vi "TIC_main.vi"() -> ()   [LabVIEW 2011]
panel:
  out "dT/dt (K / min)":dbl
  in  "setPID":bool
  in  "D":dbl
  in  "I":dbl
  in  "P":dbl
  out "Ramp in K/s":dbl
  out "Waveform Chart":dbl(graph)
  out "Ramp T (K)":dbl
  out "OldVal":dbl
  in  "Ramp (K/min)":dbl
  in  "Setpoint (K)":dbl
  in  "TIC 500":refnum<visa-resource-name>="COM6"
  out "stateMachine0":string
  in  "EXIT":bool
  in  "Valve open(V)":dbl min=0.0 max=10.0 step=0.05
  out "Valve (V)":dbl format="%.1g"
  out "Heater OUT (W)":dbl
  out "Temperature (K)":dbl
  # "T > N2: P I D\n2.064  0.016   40.516"
  # "HELIUM: P I D\n0.753  0.024   4.154"
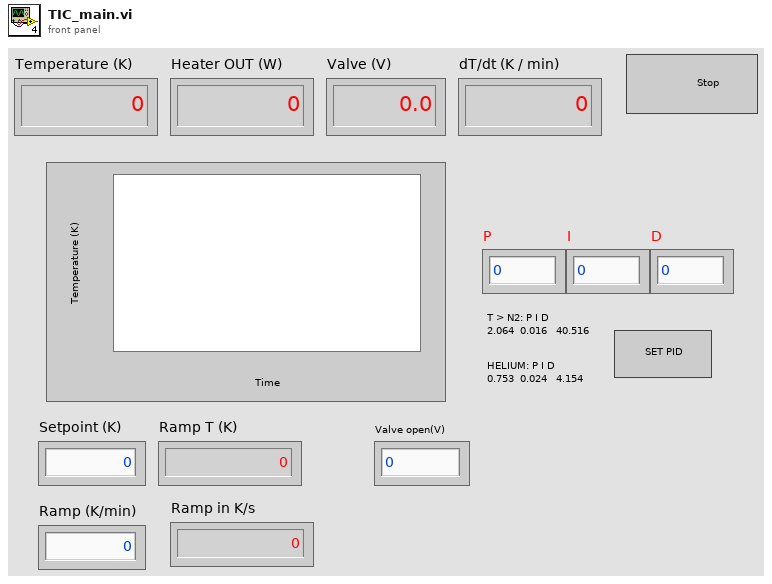
[diagram p1: front panel]
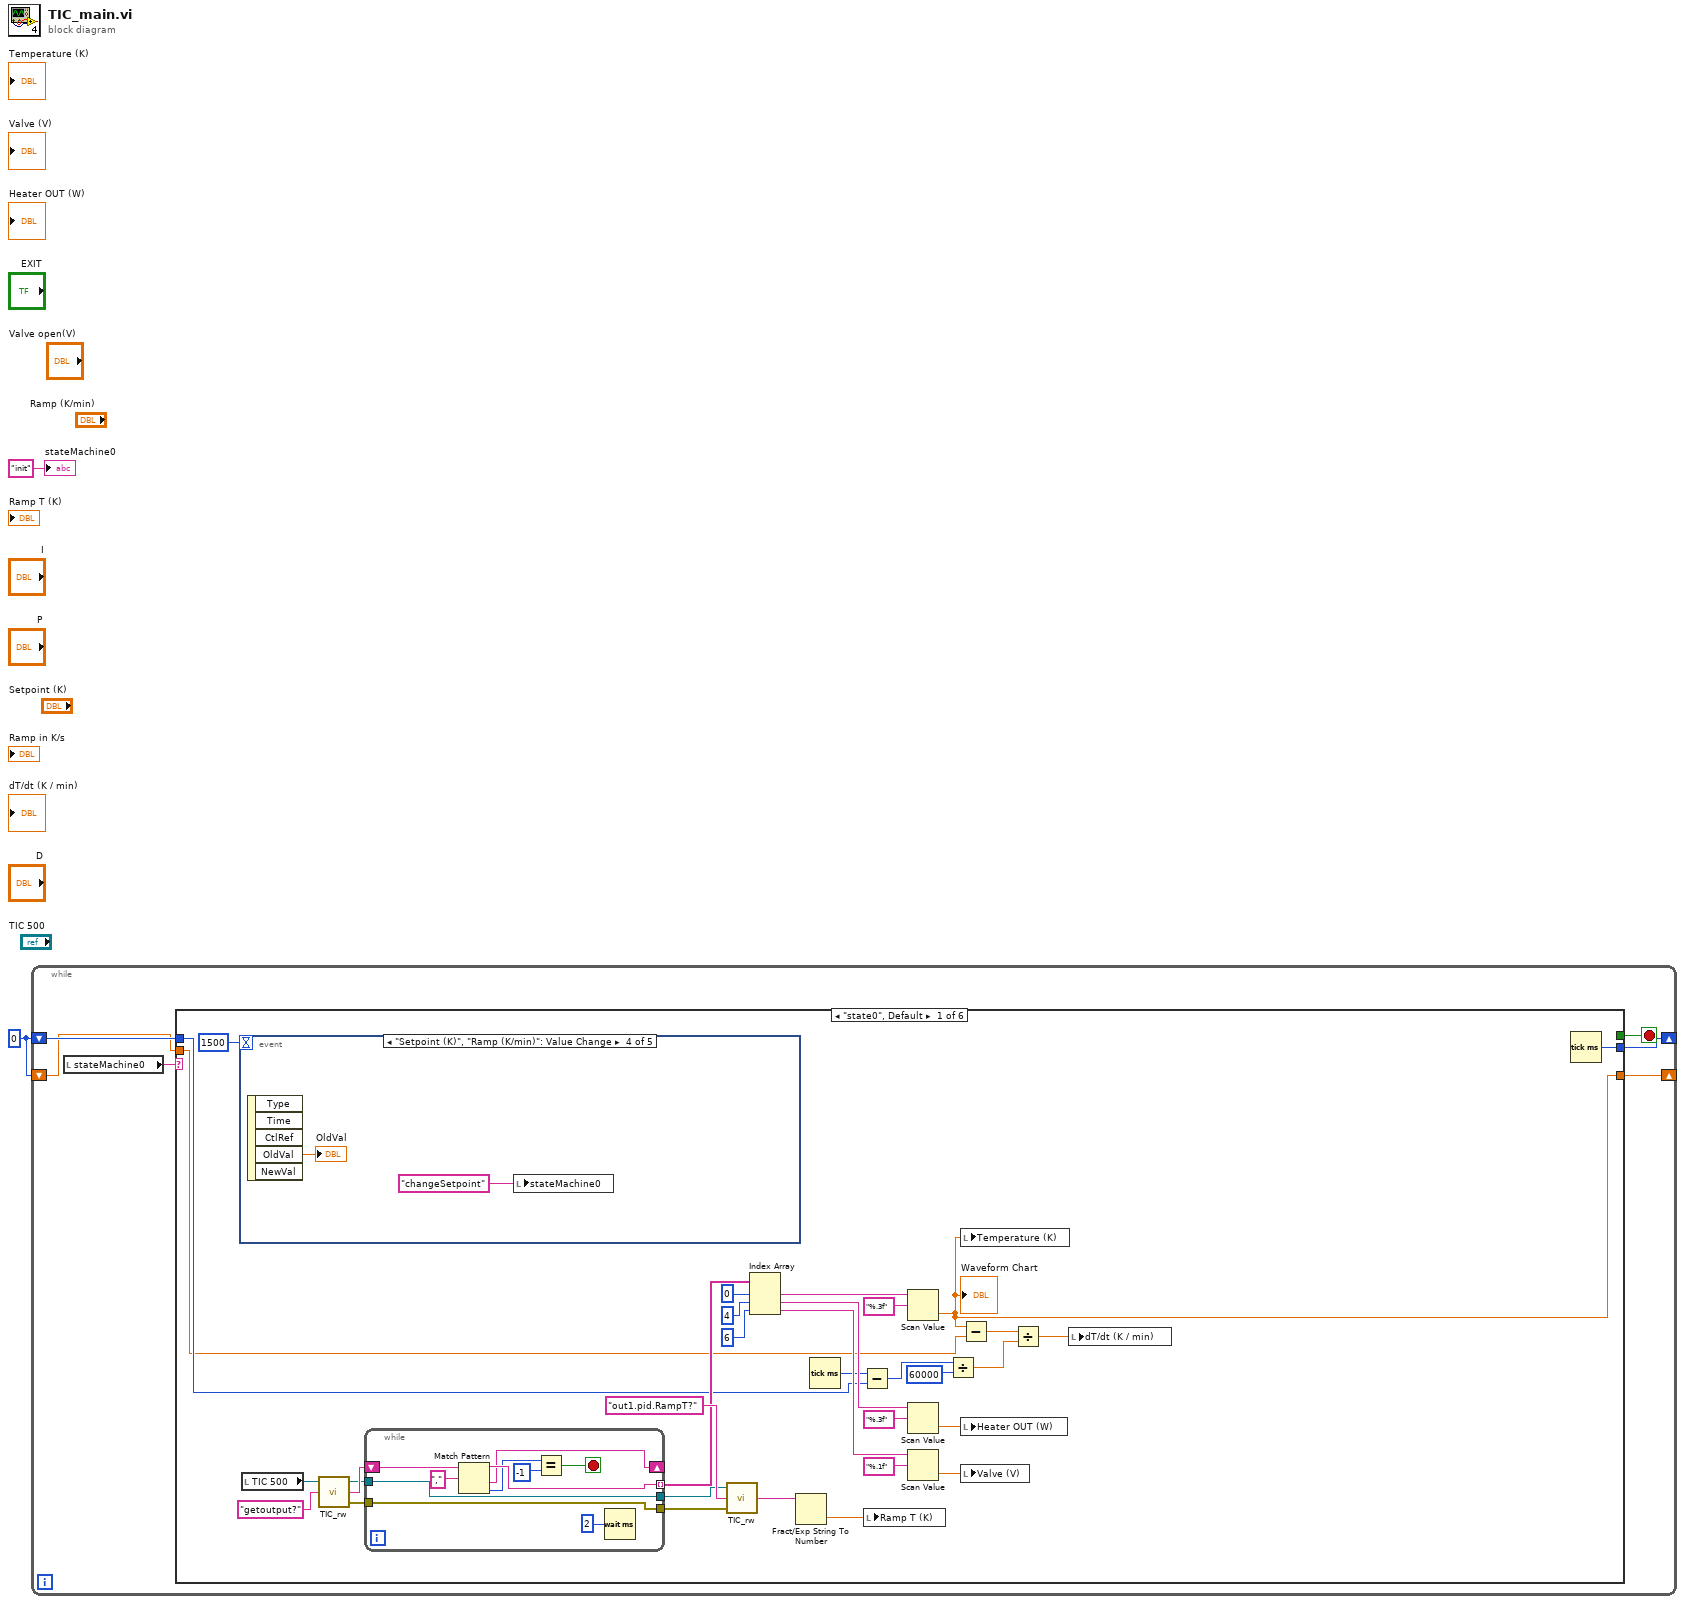
[diagram p0: block diagram]
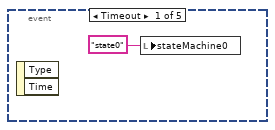
[diagram p2: hidden frame]
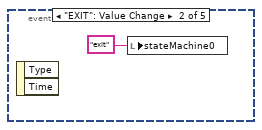
[diagram p3: hidden frame]
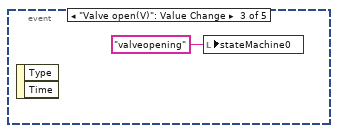
[diagram p4: hidden frame]
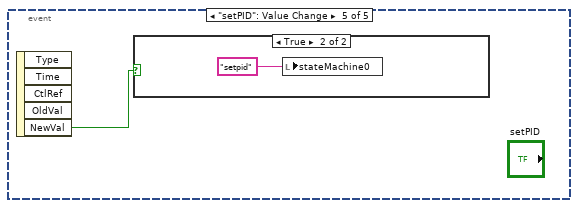
[diagram p5: hidden frame]
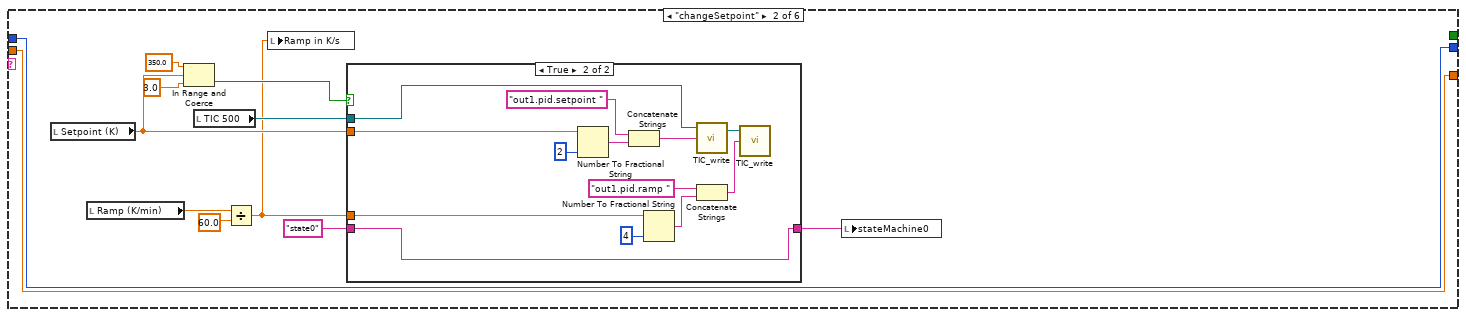
[diagram p7: hidden frame]
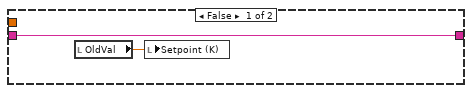
[diagram p8: hidden frame]
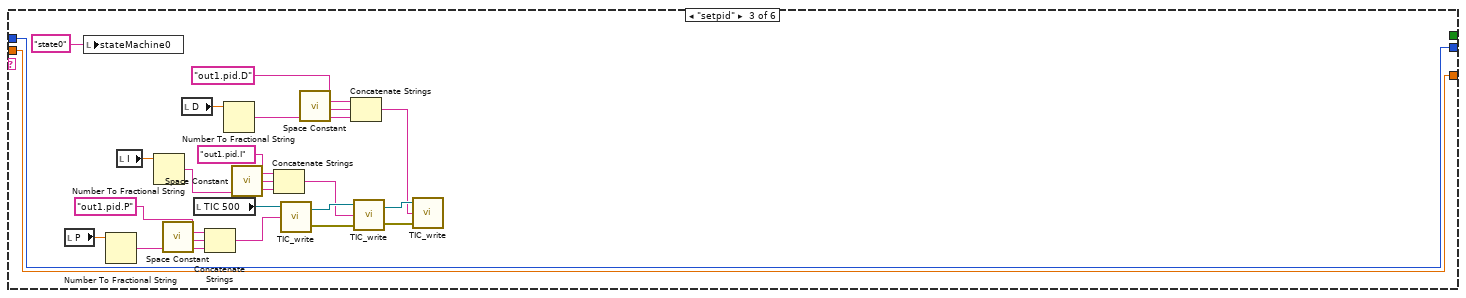
[diagram p9: hidden frame]
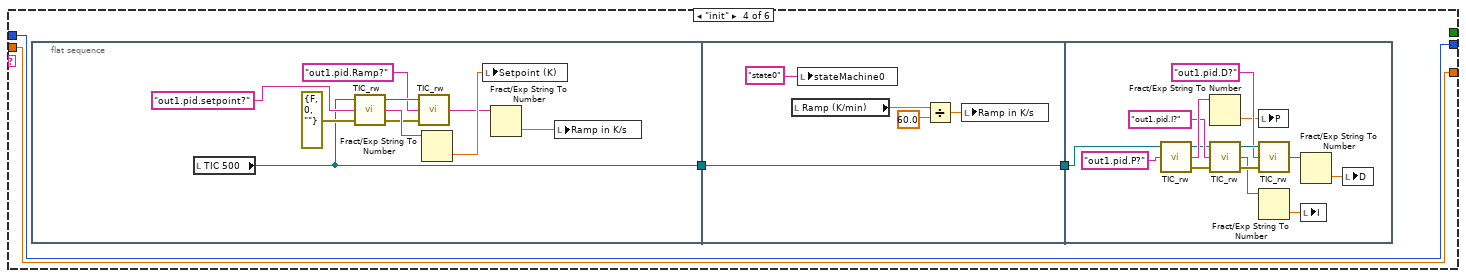
[diagram p10: hidden frame]
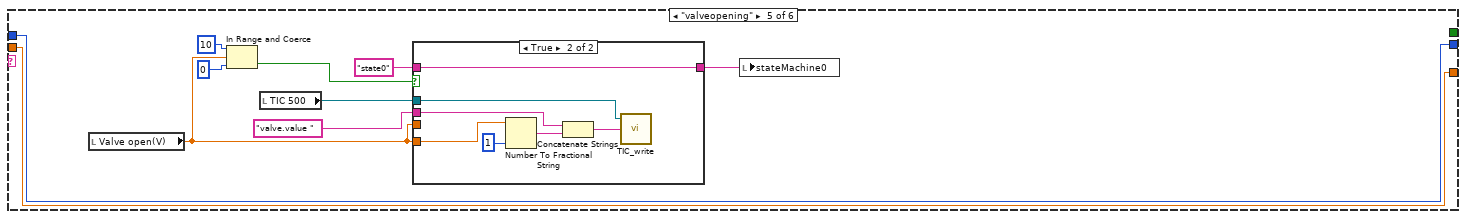
[diagram p11: hidden frame]
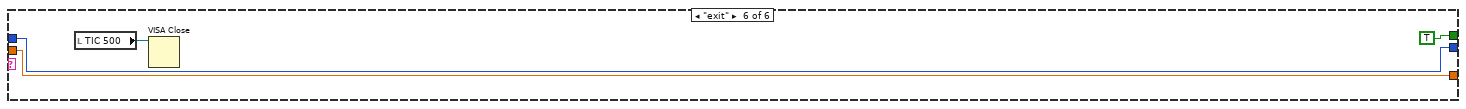
[diagram p13: hidden frame]
diagram:
  w1 = u32 0 ("millisecond timer value")
  n1 = while {
    shift-right: [w6] -> _
    shift-left: w1 -> [w5]
    shift-right: [w4] -> _
    shift-left: w1 -> [w3]
    stop <- w7 stop-if-true
    n2 = local read "stateMachine0"() -> (w8:string)
    n3 = case shown="\"state0\", Default" w8 {
      tunnel: [_ _ _ _ _ TRUE] -> w7
      tunnel: [w18 w60 w87 w109 w143 w161] -> w6
      tunnel: w5 -> [w16 w60 w87 w109 w143 w161]
      tunnel: [w10 w59 w86 w110 w142 w160] -> w4
      tunnel: w3 -> [w9 w59 w86 w110 w142 w160]
      frame "state0", Default {
        n4 = event shown="[3] \"Setpoint (K)\", \"Ramp (K/min)\": Value Change" {
          selector: _ -> [_ _ _ _ _]
          dyn-events: _ -> [_ _ _ _ _]
          timeout: 1500 -> [_ _ _ _ _]
          event Timeout {
            n5 = event-data() -> ()  [unwired: 1 in, 2 out]
            n6 = local write "stateMachine0"("state0") -> ()
          }
          event "EXIT": Value Change {
            n7 = event-data() -> ()  [unwired: 1 in, 2 out]
            n8 = local write "stateMachine0"("exit") -> ()
          }
          event "Valve open(V)": Value Change {
            n9 = event-data() -> ()  [unwired: 1 in, 2 out]
            n10 = local write "stateMachine0"("valveopening") -> ()
          }
          event "Setpoint (K)", "Ramp (K/min)": Value Change {
            n11 = event-data() -> ("OldVal"=→"OldVal":dbl)  [unwired: 1 in, 4 out]
            n12 = local write "stateMachine0"("changeSetpoint") -> ()
          }
          event "setPID": Value Change {
            n13 = event-data() -> ("NewVal"=w57:bool)  [unwired: 1 in, 4 out]
            n14 = case shown="True" w57 {
              frame False {
              }
              frame True {
                n15 = local write "stateMachine0"("setpid") -> ()
              }
            }
          }
        }
        n16 = local read "TIC 500"() -> (w40:refnum<visa-resource-name>)
        n17 = call "TIC_rw.vi"("write buffer"="getoutput?", "TIC 500"=w40) -> ("error out"=w19:errorcluster, "read buffer"=w32:string, "VISA resource name out"=w22:refnum<visa-resource-name>)  [unwired: 1 in]
        n18 = while {
          shift-right: [w48] -> _
          shift-left: w32 -> [w50]
          tunnel: [w49] -> w31 mode=indexing
          tunnel: w22 -> [w44]
          tunnel: [w44] -> w21
          tunnel: [w43] -> w20
          tunnel: w19 -> [w43]
          stop <- w45 stop-if-true
          n19 = Match Pattern(string=w50, regular expression=",") -> (before substring=w49:string, after substring=w48:string, offset past match=w47:i32)  [unwired: 1 in, 1 out]
          n20 = Equal?(x=w47, y=-1) -> (x = y?=w45:bool)
          n21 = Wait (ms)(milliseconds to wait=u32 2 ("millisecond multiple")) -> ()  [unwired: 1 out]
        }
        n22 = call "TIC_rw.vi"("error in (no error)"=w20, "write buffer"="out1.pid.RampT?", "TIC 500"=w21) -> ("read buffer"=w33:string)  [unwired: 2 out]
        n23 = Index Array(array=w31, index #1=0 ("index"), index #2=4 ("index"), index #3=6 ("index")) -> (element #1=w29:string, element #2=w27:string, element #3=w24:string)
        n24 = Fract/Exp String To Number(string=w33) -> (number=w34:dbl)  [unwired: 3 in, 1 out]
        n25 = Tick Count (ms)() -> (millisecond timer value=w17:u32)
        n26 = Subtract(x=w17, y=w16) -> (x-y=w15:u32)
        n27 = local write "Ramp T (K)"(w34) -> ()
        n28 = Scan Value(string=w29, format string="%.3f") -> (value=w10:dbl)  [unwired: 1 in, 1 out]
        "Waveform Chart" <- w10
        n29 = Scan Value(string=w27, format string="%.3f") -> (value=w26:dbl)  [unwired: 1 in, 1 out]
        n30 = Scan Value(string=w24, format string="%.1f") -> (value=w23:dbl)  [unwired: 1 in, 1 out]
        n31 = Divide(x=w15, y=u32 60000) -> (x/y=w12:dbl)
        n32 = local write "Temperature (K)"(w10) -> ()
        n33 = Subtract(x=w10, y=w9) -> (x-y=w13:dbl)
        n34 = local write "Heater OUT (W)"(w26) -> ()
        n35 = local write "Valve (V)"(w23) -> ()
        n36 = Divide(x=w13, y=w12) -> (x/y=w11:dbl)
        n37 = local write "dT/dt (K / min)"(w11) -> ()
        n38 = Tick Count (ms)() -> (millisecond timer value=w18:u32)
      }
      frame "changeSetpoint" {
        n39 = local read "Setpoint (K)"() -> (w65:dbl)
        n40 = local read "Ramp (K/min)"() -> (w62:dbl)
        n41 = In Range and Coerce(upper limit=350.0, x=w65, lower limit=3.0) -> (In Range?=w70:bool)  [unwired: 1 out]
        n42 = local read "TIC 500"() -> (w64:refnum<visa-resource-name>)
        n43 = Divide(x=w62, y=60.0) -> (x/y=w61:dbl)
        n44 = local write "Ramp in K/s"(w61) -> ()
        n45 = case shown="True" w70 {
          tunnel: "state0" -> [w72 w84]
          tunnel: [w72 w84] -> w66
          tunnel: w65 -> [_ w81]
          tunnel: w64 -> [_ w79]
          tunnel: w61 -> [_ w76]
          frame False {
            n46 = local read "OldVal"() -> (w71:dbl)
            n47 = local write "Setpoint (K)"(w71) -> ()
          }
          frame True {
            n48 = Number To Fractional String(number=w81, precision (6)=i16 2) -> (F-format string=w85:string)  [unwired: 2 in]
            n49 = Concatenate Strings("out1.pid.setpoint " ("write buffer"), w85) -> (w83:string)
            n50 = Number To Fractional String(number=w76, precision (6)=i16 4) -> (F-format string=w78:string)  [unwired: 2 in]
            n51 = call "TIC_write.vi"("write buffer"=w83, "TIC 500"=w79) -> ("VISA resource name out"=w73:refnum<visa-resource-name>)  [unwired: 1 in, 1 out]
            n52 = Concatenate Strings("out1.pid.ramp " ("write buffer"), w78) -> (w74:string)
            n53 = call "TIC_write.vi"("write buffer"=w74, "TIC 500"=w73) -> ()  [unwired: 1 in, 2 out]
          }
        }
        n54 = local write "stateMachine0"(w66) -> ()
      }
      frame "setpid" {
        n55 = local read "P"() -> (w107:dbl)
        n56 = local write "stateMachine0"("state0") -> ()
        n57 = Number To Fractional String(number=w107) -> (F-format string=w104:string)  [unwired: 3 in]
        n58 = local read "I"() -> (w97:dbl)
        n59 = Number To Fractional String(number=w97) -> (F-format string=w101:string)  [unwired: 3 in]
        n60 = call <vilib>:"Space Constant.vi"() -> ("String"=w105:string)
        n61 = local read "D"() -> (w96:dbl)
        n62 = local read "TIC 500"() -> (w95:refnum<visa-resource-name>)
        n63 = Concatenate Strings("out1.pid.P", w105, w104) -> (w94:string)
        n64 = Number To Fractional String(number=w96) -> (F-format string=w98:string)  [unwired: 3 in]
        n65 = call <vilib>:"Space Constant.vi"() -> ("String"=w102:string)
        n66 = Concatenate Strings("out1.pid.I", w102, w101) -> (w89:string)
        n67 = call "TIC_write.vi"("write buffer"=w94, "TIC 500"=w95) -> ("error out"=w93:errorcluster, "VISA resource name out"=w92:refnum<visa-resource-name>)  [unwired: 1 in]
        n68 = call <vilib>:"Space Constant.vi"() -> ("String"=w99:string)
        n69 = Concatenate Strings("out1.pid.D", w99, w98) -> (w88:string)
        n70 = call "TIC_write.vi"("error in (no error)"=w93, "write buffer"=w89, "TIC 500"=w92) -> ("error out"=w91:errorcluster, "VISA resource name out"=w90:refnum<visa-resource-name>)
        n71 = call "TIC_write.vi"("error in (no error)"=w91, "write buffer"=w88, "TIC 500"=w90) -> ()  [unwired: 2 out]
      }
      frame "init" {
        n72 = flat-sequence {
          tunnel: [w113] -> w111
          tunnel: [w123] -> w112
          tunnel: w111 -> [w123]
          tunnel: w112 -> [w136]
          frame #0 {
            n73 = local read "TIC 500"() -> (w113:refnum<visa-resource-name>)
            n74 = call "TIC_rw.vi"("error in (no error)"=errorcluster {"status"=FALSE, "code"=0, "source"=""}, "write buffer"="out1.pid.setpoint?", "TIC 500"=w113) -> ("error out"=w119:errorcluster, "read buffer"=w121:string, "VISA resource name out"=w118:refnum<visa-resource-name>)
            n75 = call "TIC_rw.vi"("error in (no error)"=w119, "write buffer"="out1.pid.Ramp?", "TIC 500"=w118) -> ("read buffer"=w116:string)  [unwired: 2 out]
            n76 = Fract/Exp String To Number(string=w121) -> (number=w120:dbl)  [unwired: 3 in, 1 out]
            n77 = local write "Setpoint (K)"(w120) -> ()
            n78 = Fract/Exp String To Number(string=w116) -> (number=w115:dbl)  [unwired: 3 in, 1 out]
            n79 = local write "Ramp in K/s"(w115) -> ()
          }
          frame #1 {
            n80 = local read "Ramp (K/min)"() -> (w126:dbl)
            n81 = local write "stateMachine0"("state0") -> ()
            n82 = Divide(x=w126, y=60.0) -> (x/y=w124:dbl)
            n83 = local write "Ramp in K/s"(w124) -> ()
          }
          frame #2 {
            n84 = call "TIC_rw.vi"("write buffer"="out1.pid.P?", "TIC 500"=w136) -> ("error out"=w138:errorcluster, "read buffer"=w140:string, "VISA resource name out"=w135:refnum<visa-resource-name>)  [unwired: 1 in]
            n85 = Fract/Exp String To Number(string=w140) -> (number=w130:dbl)  [unwired: 3 in, 1 out]
            n86 = call "TIC_rw.vi"("error in (no error)"=w138, "write buffer"="out1.pid.I?", "TIC 500"=w135) -> ("error out"=w139:errorcluster, "read buffer"=w132:string, "VISA resource name out"=w134:refnum<visa-resource-name>)
            n87 = local write "P"(w130) -> ()
            n88 = call "TIC_rw.vi"("error in (no error)"=w139, "write buffer"="out1.pid.D?", "TIC 500"=w134) -> ("read buffer"=w131:string)  [unwired: 2 out]
            n89 = Fract/Exp String To Number(string=w132) -> (number=w128:dbl)  [unwired: 3 in, 1 out]
            n90 = Fract/Exp String To Number(string=w131) -> (number=w129:dbl)  [unwired: 3 in, 1 out]
            n91 = local write "I"(w128) -> ()
            n92 = local write "D"(w129) -> ()
          }
        }
      }
      frame "valveopening" {
        n93 = local read "Valve open(V)"() -> (w147:dbl)
        n94 = In Range and Coerce(upper limit=u8 10, x=w147, lower limit=u8 0) -> (In Range?=w144:bool)  [unwired: 1 out]
        n95 = local read "TIC 500"() -> (w151:refnum<visa-resource-name>)
        n96 = case shown="True" w144 {
          tunnel: w151 -> [_ w159]
          tunnel: "valve.value " ("string") -> [_ w156]
          tunnel: w147 -> [_ _]
          tunnel: w147 -> [_ w154]
          tunnel: [w152 w153] -> w146
          tunnel: "state0" -> [w152 w153]
          frame False {
          }
          frame True {
            n97 = Number To Fractional String(number=w154, precision (6)=i16 1) -> (F-format string=w157:string)  [unwired: 2 in]
            n98 = Concatenate Strings(w156, w157) -> (w155:string)
            n99 = call "TIC_write.vi"("write buffer"=w155, "TIC 500"=w159) -> ()  [unwired: 1 in, 2 out]
          }
        }
        n100 = local write "stateMachine0"(w146) -> ()
      }
      frame "exit" {
        n101 = local read "TIC 500"() -> (w162:refnum<visa-resource-name>)
        n102 = VISA Close(VISA resource name=w162) -> ()  [unwired: 1 in, 1 out]
      }
    }
  }
  "stateMachine0" <- "init"
